vi "Set.vi"(8 "error in (no error)":errorcluster, 10 "Command":string, 11 "Handle in":i32) -> (0 "error out":errorcluster, 3 "Handle out":i32)   [LabVIEW 2013, in "Thorlabs_MC2000B.lvlib"]
uses:
  <instrlib>/Thorlabs_MC2000B/Thorlabs_MC2000B.lvlib
  <instrlib>/Thorlabs_MC2000B/Library/MC2000CommandLibWin64.dll
  <instrlib>/Thorlabs_MC2000B/Library/MC2000CommandLibWin32.dll
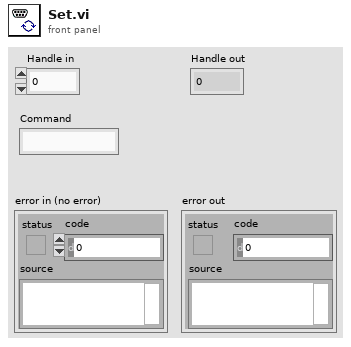
[diagram p1: front panel]
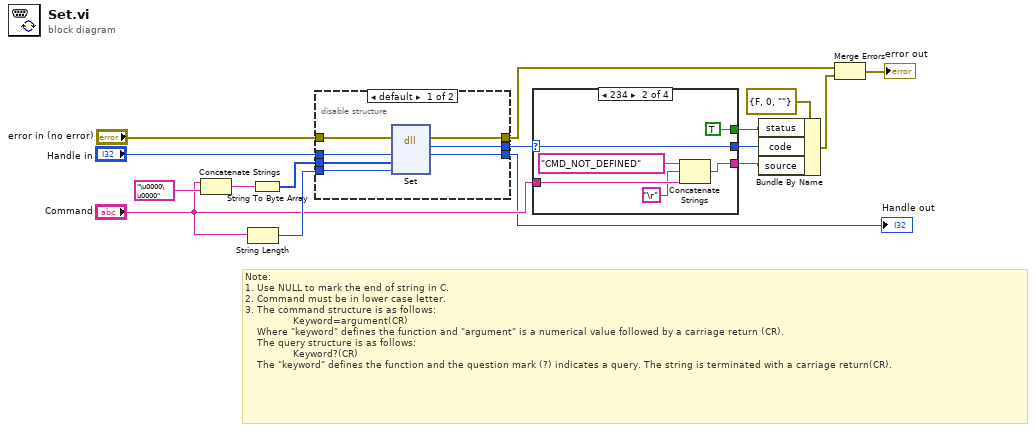
[diagram p0: block diagram]
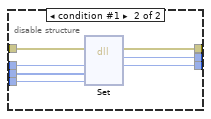
[diagram p2: hidden frame]
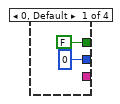
[diagram p3: hidden frame]
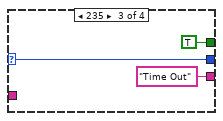
[diagram p4: hidden frame]
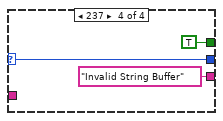
[diagram p5: hidden frame]
diagram:
  # "Note:\n1. Use NULL to mark the end of string in C.\n2. Command must be in lower case letter.\n3. The command structure is as follows:\n                Keyword=argument(CR)\n    Where \"keyword\" defines the function and \"argument\" is a numerical value followed by a carriage return (CR).\n    The query structure is as follows:\n                Keyword?(CR)\n    The \"keyword\" defines the function and the question mark (?) indicates a query. The string is terminated with a carriage return(CR)."
  n1 = Concatenate Strings("Command", "\u0000\u0000") -> (w5:string)
  n2 = String Length(string="Command") -> (length=w4:i32)
  n3 = String To Byte Array(string=w5) -> (unsigned byte array=w15:u8[])
  n4 = disable-structure shown="default" {
    disable-tunnel: w15 -> [w23 w30]
    disable-tunnel: [w22 w29] -> w14
    disable-tunnel: "error in (no error)" -> [w21 w28]
    disable-tunnel: [w20 w27] -> w8
    disable-tunnel: w4 -> [w19 w26]
    disable-tunnel: "Handle in" -> [w18 w25]
    disable-tunnel: [w17 w24] -> w1
    frame condition #0 (active) {
      n5 = dll-call lib="C:/Program Files (x86)/National Instruments/LabVIEW 2013/instr.lib/Thorlabs_MC2000B/Library/MC2000CommandLibWin32.dll" fn="Set"(error in=w21, "Handle"=w18, "Command"=w23, "Length"=w19) -> (error out=w20:errorcluster, "return type"=w22:i32, "Handle"=w17:i32)  [unwired: 4 in, 1 out]
    }
    frame condition #1 {
      n6 = dll-call lib="D:/Program Files/National Instruments/LabVIEW 2011/instr.lib/Thorlabs_MC2000B/Library/MC2000CommandLibWin64.dll" fn="Set"(error in=w28, "Handle"=w25, "Command"=w30, "Length"=w26) -> (error out=w27:errorcluster, "return type"=w29:i32, "Handle"=w24:i32)  [unwired: 4 in, 1 out]
    }
  }
  "Handle out" <- w1
  n7 = case shown="234" w14 {
    selector: w14 -> [_ w37 w39 w42]
    tunnel: [_ w36 "Time Out" "Invalid String Buffer"] -> w9
    tunnel: [FALSE TRUE TRUE TRUE] -> w11
    tunnel: [0 w37 w39 w42] -> w10
    tunnel: "Command" -> [_ w34 _ _]
    frame 0, Default {
    }
    frame 234 {
      n8 = Concatenate Strings("CMD_NOT_DEFINED", "\r", w34) -> (w36:string)
    }
    frame 235 {
    }
    frame 237 {
    }
  }
  n9 = Bundle By Name(cluster=errorcluster {"status"=FALSE, "code"=0, "source"=""} ("error out"), "status"=w11, "code"=w10, "source"=w9) -> (w7:errorcluster)
  n10 = Merge Errors(w8, w7) -> (→"error out":errorcluster)
